vi "Decay  Data Analysis.vi"() -> ()   [LabVIEW 2015]
uses:
  <vilib>/Utility/file.llb/Read Delimited Spreadsheet (DBL).vi
  <vilib>/Analysis/NI_AALPro.lvlib
panel:
  out "Constant Rate":dbl[][](graph) caption="Histogram"
  out "Decay Rate":cluster{"all rows":dbl[], "all rows":dbl[]}[](graph)
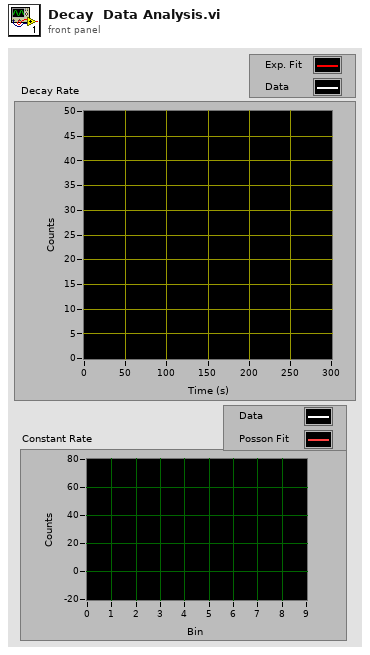
[diagram p1: front panel]
types:
  T1 = cluster{"all rows":dbl[], "Best Exponential Fit":dbl[]}
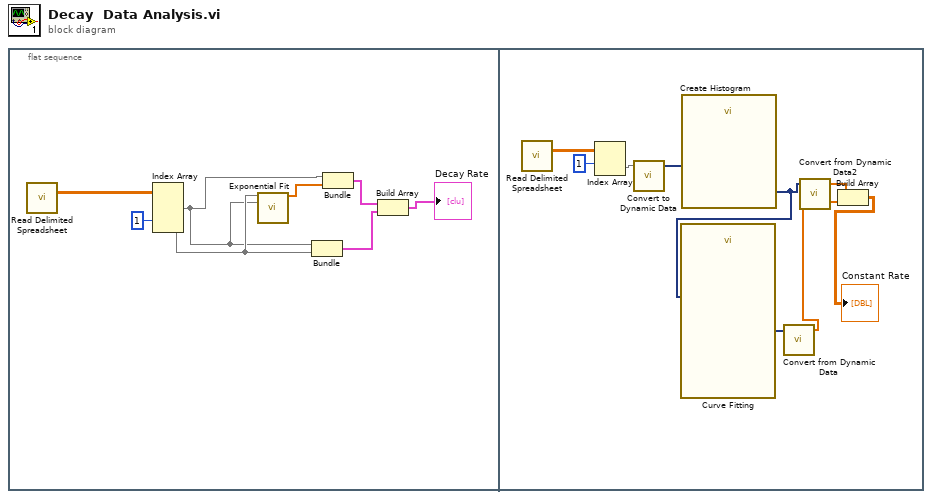
[diagram p0: block diagram]
diagram:
  n1 = flat-sequence {
    frame #0 {
      n2 = call-poly <vilib>:"Read Delimited Spreadsheet.vi"() -> ("all rows"=w7:dbl[][])  [unwired: 10 in, 5 out]
      n3 = Index Array(array=w7, index (row) #2=1 ("index (row)")) -> (element #1=w1:dbl[], element #2=w3:dbl[])  [unwired: 3 in]
      n4 = call <vilib>:"Exponential Fit.vi"("Y"=w3, "X"=w1) -> ("Best Exponential Fit"=w6:dbl[])  [unwired: 8 in, 5 out]
      n5 = Bundle("all rows"=w1, "all rows"=w3) -> (w5:cluster{"all rows":dbl[], "all rows":dbl[]})  [unwired: 1 in]
      n6 = Bundle("all rows"=w1, "Best Exponential Fit"=w6) -> (w2:T1)  [unwired: 1 in]
      n7 = Build Array(w2, w5) -> (→"Decay Rate":cluster{"all rows":dbl[], "all rows":dbl[]}[])
    }
    frame #1 {
      n8 = call-poly <vilib>:"Read Delimited Spreadsheet.vi"() -> ("all rows"=w17:dbl[][])  [unwired: 10 in, 5 out]
      n9 = Index Array(array=w17, index (row)=1) -> (element=w14:dbl[])  [unwired: 1 in]
      n10 = call "Convert to Dynamic Data"("Array"=w14) -> ("Dynamic Data Type"=w15:dynamicdata)  [unwired: 3 in]
      n11 = call "Create Histogram"("Signal"=w15) -> ("Histogram"=w11:dynamicdata)  [unwired: 9 in, 1 out]
      n12 = call "Curve Fitting"("Signals"=w11) -> ("best fit"=w13:dynamicdata)  [unwired: 6 in, 4 out]
      n13 = call "Convert from Dynamic Data"("Dynamic Data Type"=w13) -> ("Array"=w12:dbl[])  [unwired: 3 in]
      n14 = call "Convert from Dynamic Data2"("Dynamic Data Type"=w11) -> ("Array"=w10:dbl[])  [unwired: 3 in]
      n15 = Build Array(w10, w12) -> (→"Constant Rate":dbl[][])
    }
  }
